vi "ReadFileDialog.vi"(6 "File Text":string, 8 "error in (no error)":errorcluster, 9 "File name":string, 10 "Console in":string, 11 "Python in":T1) -> (0 "error out":errorcluster, 2 "Console":string)   [LabVIEW 2022 SP3]
uses:
  PythonCtrl.ctl
  Processors.ctl
  <vilib>/Utility/error.llb/Trim Whitespace One-Sided.vi
panel:
  out "diff":i16
  out "File received":string
  out "File Sent":string
  in  "Done":bool
  in  "Abort":bool
  out "Python out":T1
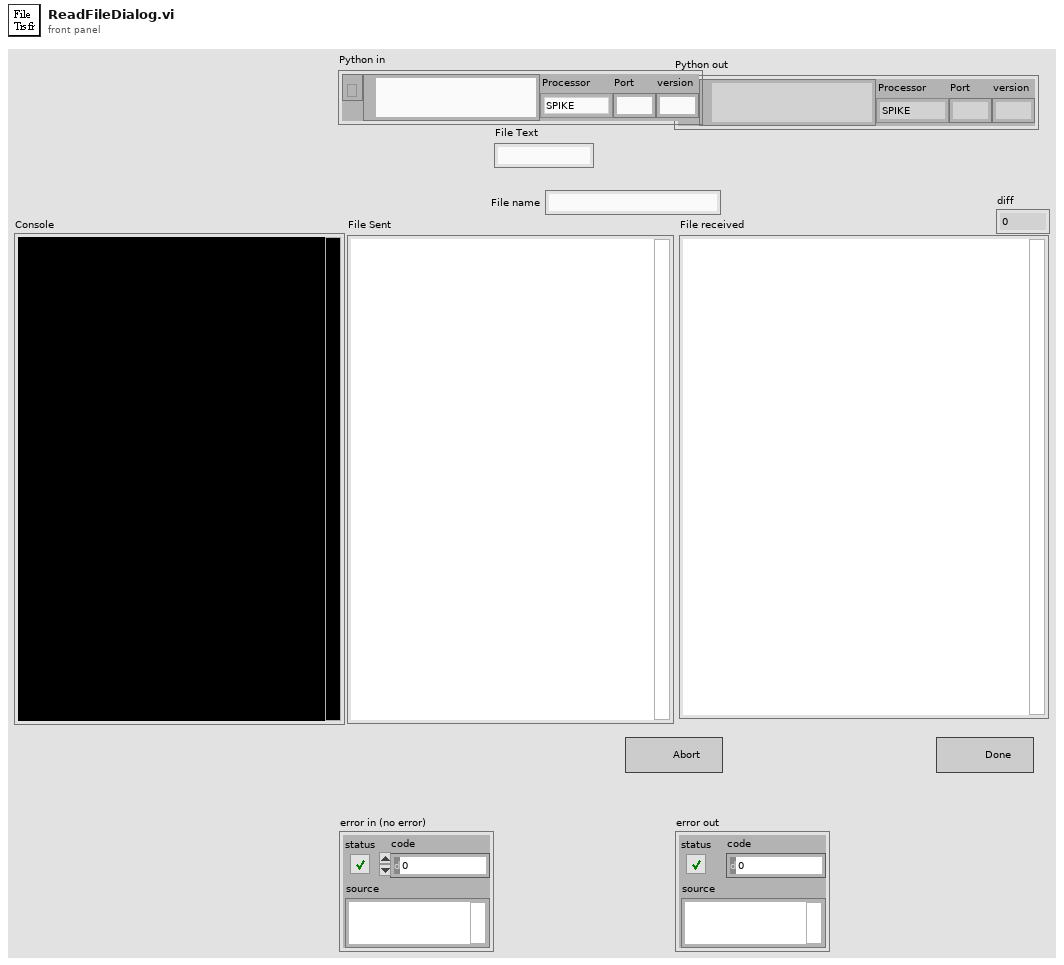
[diagram p1: front panel]
types:
  T1 = typedef "PythonCtrl.ctl" = cluster{"session":refnum<k35>, "PyPath":path, "Processor":T2, "Port":string, "version":string}
  T2 = typedef "Processors.ctl" = enum16{"SPIKE", "Pi", "Pi_ssh", "OpenMV", "Dunio"}
  T3 = enum16{"read", "write pause", "write port", "write path", "write all"}
  T4 = enum32{"Invalid", "Standard", "Closed", "Hidden", "Minimized", "Maximized"}
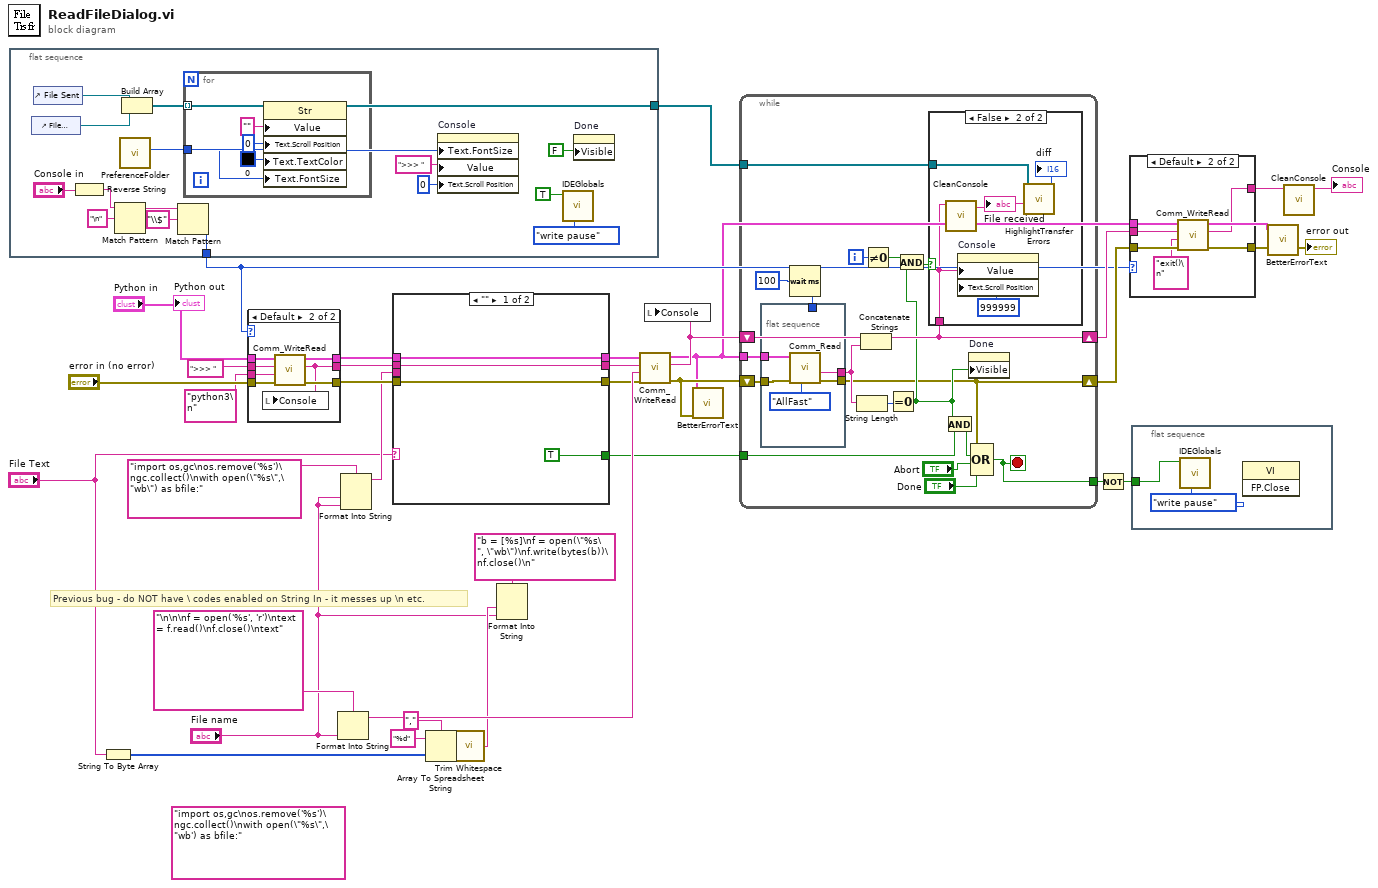
[diagram p0: block diagram]
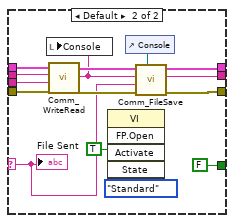
[diagram p4: hidden frame]
diagram:
  (unwired) "import os,gc\nos.remove('%s')\ngc.collect()\nwith open(\"%s\",\"wb') as bfile:" ("function name")
  # "Previous bug - do NOT have \\ codes enabled on String In - it messes up \\n etc."
  n1 = flat-sequence {
    tunnel: [w48] -> w18
    tunnel: [w39] -> w12
    frame #0 {
      n2 = control-ref of="File received"() -> (w49:refnum<vi>)
      n3 = control-ref of="File Sent"() -> (w50:refnum<vi>)
      n4 = Reverse String(1:"Console in") -> (0:w43:string)
      n5 = Match Pattern(string=w43, regular expression="\n") -> (before substring=w44:string)  [unwired: 1 in, 3 out]
      n6 = call "PreferenceFolder.vi"() -> ("FontSize"=w38:u8)  [unwired: 4 in, 7 out]
      n7 = Build Array(w50, w49) -> (w48:refnum<vi>[])
      n8 = Match Pattern(string=w44, regular expression="\\$") -> (offset past match=w39:i32)  [unwired: 1 in, 3 out]
      n9 = for {
        tunnel: w48 -> [w55] mode=indexing
        tunnel: w38 -> [w51]
        n10 = property on="Property Node" class="Str"(reference=w55, "Value"="", "Text.Scroll Position"=u32 0, "Text.TextColor"=u32 0 ("Text.Text Colors:Text Color"), "Text.FontSize"=w51) -> ()  [unwired: 1 in, 2 out]
      }
      n11 = property on="Console" class="Str"("Text.FontSize"=w38, "Value"=">>> " ("Console"), "Text.Scroll Position"=u32 0) -> ()  [unwired: 2 in, 2 out]
      n12 = call "IDEGlobals.vi"("task"=T3."write pause", "pause?"=TRUE) -> ()  [unwired: 7 in, 3 out]
      n13 = property on="Done" class="Bool"("Visible"=FALSE) -> ()  [unwired: 2 in, 2 out]
    }
  }
  n14 = String To Byte Array(string="File Text") -> (unsigned byte array=w6:u8[])
  n15 = case shown="Default" w12 {
    tunnel: [w56 w65] -> w27
    tunnel: [w57 w59] -> w26
    tunnel: [w58 w64] -> w25
    tunnel: "Python in" -> [w58 w63]
    tunnel: ">>> " ("Text to write") -> [w57 w62]
    tunnel: "error in (no error)" -> [w56 w61]
    tunnel: "python3\n" ("regular expression") -> [_ w60]
    frame -1 {
    }
    frame Default {
      n16 = call "Comm_WriteRead.vi"("error in (no error)"=w61, "Code"=w60, "Console In"=w62, "Python"=w63) -> ("error out"=w65:errorcluster, "Console"=w59:string, "Python"=w64:T1)  [unwired: 5 in]
      n17 = local write "Console"(w59) -> ()
    }
  }
  n18 = Format Into String(format string="\n\n\nf = open('%s', 'r')\ntext = f.read()\nf.close()\ntext" ("function name"), "File name") -> (resulting string=w35:string)  [unwired: 2 in, 1 out]
  n19 = Format Into String(format string="import os,gc\nos.remove('%s')\ngc.collect()\nwith open(\"%s\",\"wb\") as bfile:" ("function name"), "File name", "File name") -> (resulting string=w13:string)  [unwired: 2 in, 1 out]
  n20 = case shown="\"\"" "File Text" {
    selector: "File Text" -> [_ w70]
    tunnel: [w67 w75] -> w32
    tunnel: [w68 w73] -> w31
    tunnel: [w69 w74] -> w30
    tunnel: w25 -> [w69 w82]
    tunnel: w26 -> [w68 w83]
    tunnel: w27 -> [w67 w84]
    tunnel: [TRUE FALSE] -> w17
    tunnel: w13 -> [_ w80]
    frame "" {
    }
    frame Default {
      n21 = call "Comm_WriteRead.vi"("error in (no error)"=w84, "Code"=w80, "Console In"=w83, "Python"=w82) -> ("error out"=w76:errorcluster, "Console"=w72:string, "Python"=w77:T1)  [unwired: 5 in]
      n22 = local write "Console"(w72) -> ()
      n23 = invoke class="VI" method="FP.Open"("Activate"=TRUE ("Activate?"), "State"=T4."Standard") -> ()  [unwired: 3 in, 5 out]
      n24 = control-ref of="Console"() -> (w71:refnum<vi>)
      n25 = call "Comm_FileSave.vi"("Console"=w71, "error in (no error)"=w76, "Code"=w70, "Console In"=w72, "Python"=w77) -> ("error out"=w75:errorcluster, "Console"=w73:string, "Python"=w74:T1)  [unwired: 4 in]
      "File Sent" <- w70
    }
  }
  n26 = Array To Spreadsheet String(delimiter (Tab)=",", array=w6, 3:"%d" ("format string")) -> (spreadsheet string=w3:string)
  n27 = call <vilib>:"Trim Whitespace.vi"("string"=w3) -> ("trimmed string"=w2:string)  [unwired: 1 in]
  n28 = Format Into String(format string="b = [%s]\nf = open(\"%s\", \"wb\")\nf.write(bytes(b))\nf.close()\n" ("function name"), w2, "File name") -> ()  [unwired: 2 in, 2 out]
  n29 = call "Comm_WriteRead.vi"("error in (no error)"=w32, "Code"=w35, "Console In"=w31, "Python"=w30) -> ("error out"=w9:errorcluster, "Console"=w29:string, "Python"=w8:T1)  [unwired: 5 in]
  n30 = local write "Console"(w29) -> ()
  n31 = call "BetterErrorText.vi"("error in (no error)"=w9, "Python"=w8) -> ()  [unwired: 8 in, 2 out]
  n32 = while {
    shift-right: [w99] -> w19
    shift-left: w29 -> [w102]
    tunnel: w8 -> [w100]
    shift-right: [w86] -> w20
    shift-left: w9 -> [w103]
    tunnel: [w95] -> w28
    tunnel: w18 -> [w94]
    tunnel: w17 -> [w93]
    i -> [w89]
    stop <- w95 stop-if-true
    n33 = flat-sequence {
      tunnel: w103 -> [w108]
      tunnel: [w107] -> w101
      tunnel: w100 -> [w106]
      tunnel: [w105] -> w86
      tunnel: w85 -> [_]
      frame #0 {
        n34 = call "Comm_Read.vi"("Task"=enum16{"Instant", "All", "AllFast", "Params"}."AllFast", "error in (no error)"=w108, "Python"=w106) -> ("error out"=w105:errorcluster, "Text read"=w107:string)  [unwired: 7 in]
      }
    }
    n35 = Wait (ms)(milliseconds to wait=u32 100) -> (millisecond timer value=w85:u32)
    n36 = String Length(string=w101) -> (length=w96:i32)
    n37 = Concatenate Strings(w102, w101) -> (w99:string)
    n38 = Not Equal To 0?(x=w89) -> (x != 0?=w90:bool)
    n39 = Equal To 0?(x=w96) -> (x = 0?=w88:bool)
    n40 = And(x=w90, y=w88) -> (x .and. y?=w87:bool)
    n41 = case shown="False" w87 {
      tunnel: w99 -> [_ w112]
      tunnel: w94 -> [_ w111]
      frame True {
      }
      frame False {
        n42 = call "CleanConsole.vi"("Console in"=w112) -> ("Console out"=w109:string)  [unwired: 10 in]
        "File received" <- w109
        n43 = property on="Console" class="Str"("Value"=w112, "Text.Scroll Position"=u32 999999) -> ()  [unwired: 2 in, 2 out]
        n44 = call "HighlightTransferErrors.vi"("File received"=w109, "Sent/Recieved"=w111) -> ("diff"=→"diff":i16)  [unwired: 9 in]
      }
    }
    n45 = And(x=w88, y=w93) -> (x .and. y?=w92:bool)
    n46 = property on="Done" class="Bool"("Visible"=w88) -> ()  [unwired: 2 in, 2 out]
    n47 = Compound Arithmetic op=OR(w86, w92, "Abort", "Done") -> (w95:bool)
  }
  n48 = Not(x=w28) -> (.not. x?=w11:bool)
  n49 = case shown="Default" w12 {
    tunnel: [w115 w121] -> w10
    tunnel: w8 -> [_ w120]
    tunnel: w19 -> [w114 w119]
    tunnel: w20 -> [w115 w118]
    tunnel: [w114 w116] -> w16
    frame -1 {
    }
    frame Default {
      n50 = call "Comm_WriteRead.vi"("error in (no error)"=w118, "Code"="exit()\n" ("regular expression"), "Console In"=w119, "Python"=w120) -> ("error out"=w121:errorcluster, "Console"=w116:string)  [unwired: 5 in, 1 out]
    }
  }
  "error out" <- w10
  n51 = flat-sequence {
    tunnel: w11 -> [w122]
    frame #0 {
      n52 = call "IDEGlobals.vi"("task"=T3."write pause", "pause?"=w122) -> ()  [unwired: 7 in, 3 out]
      n53 = invoke class="VI" method="FP.Close"() -> ()  [unwired: 3 in, 3 out]
    }
  }
  n54 = call "BetterErrorText.vi"("error in (no error)"=w10, "Python"=w8) -> ()  [unwired: 8 in, 2 out]
  n55 = call "CleanConsole.vi"("Console in"=w16) -> ("Console out"=→"Console":string)  [unwired: 10 in]
  "Python out" <- "Python in"
